vi "Format View Parameter.vi"(9 "Column":T1, 11 "VI Data":T2) -> (2 "View Parameter":string)   [LabVIEW 2020, in "VI Properties Editor.lvlib"]
doc: "Formats the parameter specified by <B>Column</B> into a string value to be used in filter and sort functions."
uses:
  VI Properties Editor.lvlib
  CTLs/VI Data.ctl
  CTLs/VI Properties.ctl
  <vilib>/picture/picture.llb/imagedata.ctl
  CTLs/Control Properties.ctl
  CTLs/Column Name.ctl
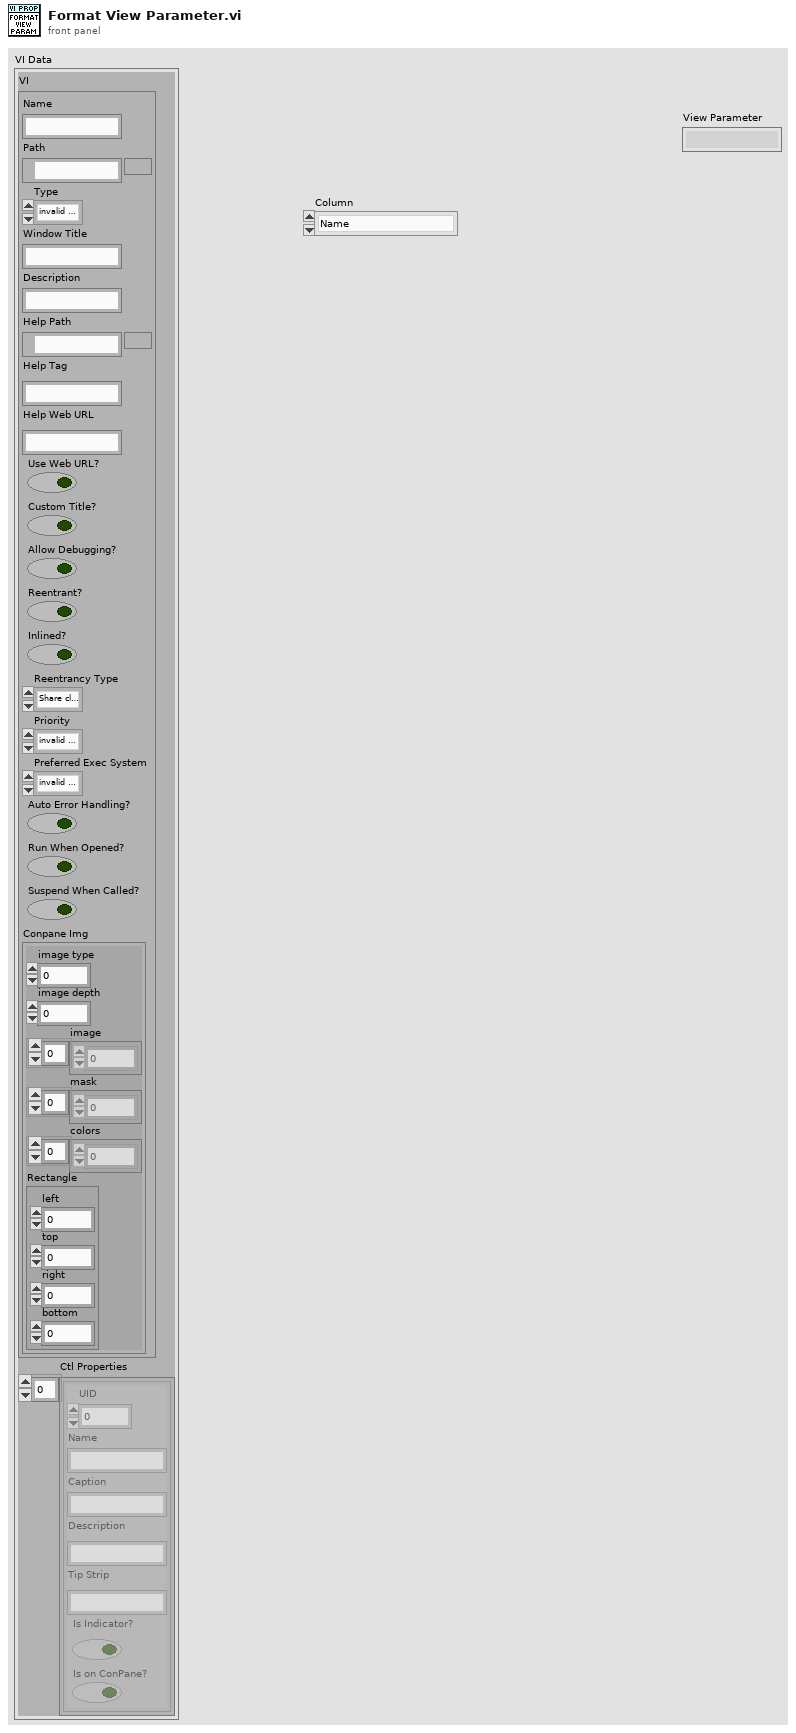
[diagram p1: front panel]
types:
  T1 = typedef "VI Properties Editor.lvlib/Column Name.ctl" = enum16{"Name", "Path", "Type", "Window Title", "Description", "Help Path", "Help Tag", "Custom Title?", "Reentrancy", "Inlined?", "Help URL", "Help Type", "Allow Debugging?", "Auto Error Handling?", "Run When Opened?", "Suspend When Called?", "Priority", "Preferred Exec Sytem"}
  T2 = typedef "VI Properties Editor.lvlib/VI Data.ctl" = cluster{"VI":T3, "Ctl Properties":T5[]}
  T3 = typedef "VI Properties Editor.lvlib/VI Properties.ctl" = cluster{"Name":string, "Path":path, "Type":enum32{"invalid VI type", "Standard VI", "Control VI", "Global VI", "Polymorphic VI", "Configuration VI", "SubSystem", "Facade VI", "Method VI", "Statechart Diagram VI"}, "Window Title":string, "Description":string, "Help Path":path, "Help Tag":string, "Help Web URL":string, "Use Web URL?":bool, "Custom Title?":bool, "Allow Debugging?":bool, "Reentrant?":bool, "Inlined?":bool, "Reentrancy Type":enum16{"Share clones between instances", "Preallocate clone for each instance"}, "Priority":enum32{"invalid priority", "background priority", "normal priority", "above normal priority", "high priority", "time critical priority", "subroutine"}, "Preferred Exec System":enum32{"invalid execution system", "user interface", "standard", "instrument i/o", "data acquisition", "other 1", "other 2", "same as caller"}, "Auto Error Handling?":bool, "Run When Opened?":bool, "Suspend When Called?":bool, "Conpane Img":T4}
  T4 = typedef "imagedata.ctl" = cluster{"image type":i32, "image depth":i32, "image":u8[], "mask":u8[], "colors":u32[], "Rectangle":cluster{"left":i16, "top":i16, "right":i16, "bottom":i16}}
  T5 = typedef "VI Properties Editor.lvlib/Control Properties.ctl" = cluster{"UID":i32, "Name":string, "Caption":string, "Description":string, "Tip Strip":string, "Is Indicator?":bool, "Is on ConPane?":bool}
  T6 = enum32{"invalid VI type", "Standard VI", "Control VI", "Global VI", "Polymorphic VI", "Configuration VI", "SubSystem", "Facade VI", "Method VI", "Statechart Diagram VI"}
  T7 = enum16{"Share clones between instances", "Preallocate clone for each instance"}
  T8 = enum32{"invalid priority", "background priority", "normal priority", "above normal priority", "high priority", "time critical priority", "subroutine"}
  T9 = enum32{"invalid execution system", "user interface", "standard", "instrument i/o", "data acquisition", "other 1", "other 2", "same as caller"}
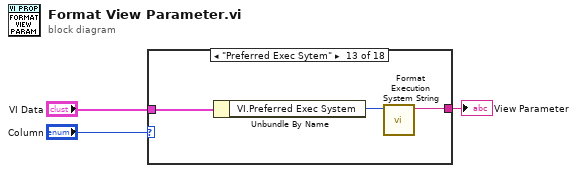
[diagram p0: block diagram]
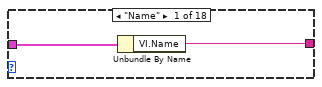
[diagram p2: hidden frame]
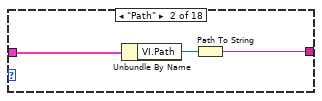
[diagram p3: hidden frame]
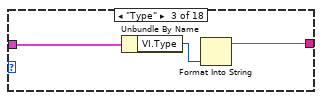
[diagram p4: hidden frame]
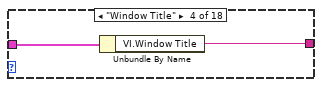
[diagram p5: hidden frame]
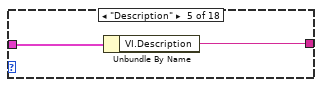
[diagram p6: hidden frame]
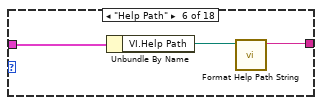
[diagram p7: hidden frame]
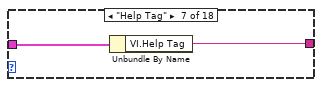
[diagram p8: hidden frame]
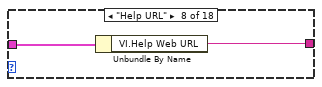
[diagram p9: hidden frame]
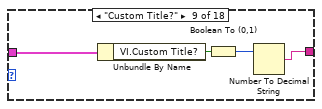
[diagram p10: hidden frame]
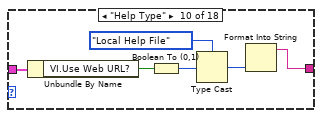
[diagram p11: hidden frame]
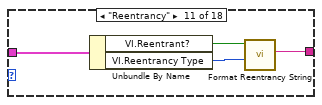
[diagram p12: hidden frame]
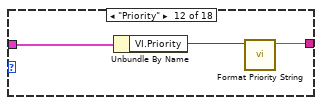
[diagram p13: hidden frame]
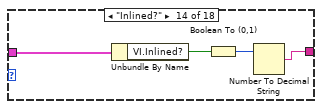
[diagram p14: hidden frame]
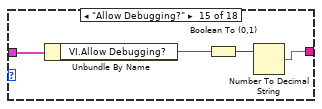
[diagram p15: hidden frame]
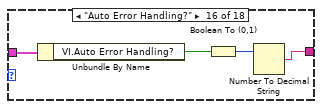
[diagram p16: hidden frame]
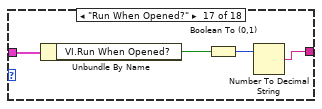
[diagram p17: hidden frame]
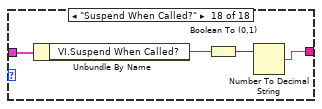
[diagram p18: hidden frame]
diagram:
  n1 = case shown="\"Preferred Exec Sytem\"" "Column" {
    tunnel: "VI Data" -> [w5 w8 w11 w13 w15 w18 w20 w22 w26 w32 w36 w39 w42 w46 w50 w54 w58 w62]
    tunnel: [w4 w6 w10 w12 w14 w17 w19 w21 w23 w27 w34 w38 w40 w43 w47 w51 w55 w59] -> w1
    frame "Name" {
      n2 = Unbundle By Name(w5) -> ("VI.Name"=w4:string)
    }
    frame "Path" {
      n3 = Unbundle By Name(w8) -> ("VI.Path"=w7:path)
      n4 = Path To String(path=w7) -> (string=w6:string)
    }
    frame "Type" {
      n5 = Unbundle By Name(w11) -> ("VI.Type"=w9:T6)
      n6 = Format Into String(w9) -> (resulting string=w10:string)  [unwired: 3 in, 1 out]
    }
    frame "Window Title" {
      n7 = Unbundle By Name(w13) -> ("VI.Window Title"=w12:string)
    }
    frame "Description" {
      n8 = Unbundle By Name(w15) -> ("VI.Description"=w14:string)
    }
    frame "Help Path" {
      n9 = Unbundle By Name(w18) -> ("VI.Help Path"=w16:path)
      n10 = call "Format Help Path String.vi"("Help Path"=w16) -> ("Help Path String"=w17:string)  [unwired: 10 in]
    }
    frame "Help Tag" {
      n11 = Unbundle By Name(w20) -> ("VI.Help Tag"=w19:string)
    }
    frame "Help URL" {
      n12 = Unbundle By Name(w22) -> ("VI.Help Web URL"=w21:string)
    }
    frame "Custom Title?" {
      n13 = Unbundle By Name(w26) -> ("VI.Custom Title?"=w25:bool)
      n14 = Boolean To (0,1)(Boolean=w25) -> (0, 1=w24:i16)
      n15 = Number To Decimal String(number=w24) -> (decimal integer string=w23:string)  [unwired: 1 in]
    }
    frame "Help Type" {
      n16 = Unbundle By Name(w32) -> ("VI.Use Web URL?"=w31:bool)
      n17 = Boolean To (0,1)(Boolean=w31) -> (0, 1=w30:i16)
      n18 = Type Cast(type=enum16{"Local Help File", "Web-based Help"}."Local Help File" ("FP.Help Type"), x=w30) -> (*(type *) &x=w28:enum16{"Local Help File", "Web-based Help"})
      n19 = Format Into String(w28) -> (resulting string=w27:string)  [unwired: 3 in, 1 out]
    }
    frame "Reentrancy" {
      n20 = Unbundle By Name(w36) -> ("VI.Reentrant?"=w33:bool, "VI.Reentrancy Type"=w35:T7)
      n21 = call "Format Reentrancy String.vi"("Reentrancy Type"=w35, "Reentrant?"=w33) -> ("Reentrancy String"=w34:string)  [unwired: 9 in]
    }
    frame "Priority" {
      n22 = Unbundle By Name(w39) -> ("VI.Priority"=w37:T8)
      n23 = call "Format Priority String.vi"("Priority"=w37) -> ("Priority String"=w38:string)  [unwired: 10 in]
    }
    frame "Preferred Exec Sytem" {
      n24 = Unbundle By Name(w42) -> ("VI.Preferred Exec System"=w41:T9)
      n25 = call "Format Execution System String.vi"("Preferred Exec System"=w41) -> ("Preferred Exec System String"=w40:string)  [unwired: 10 in]
    }
    frame "Inlined?" {
      n26 = Unbundle By Name(w46) -> ("VI.Inlined?"=w45:bool)
      n27 = Boolean To (0,1)(Boolean=w45) -> (0, 1=w44:i16)
      n28 = Number To Decimal String(number=w44) -> (decimal integer string=w43:string)  [unwired: 1 in]
    }
    frame "Allow Debugging?" {
      n29 = Unbundle By Name(w50) -> ("VI.Allow Debugging?"=w49:bool)
      n30 = Boolean To (0,1)(Boolean=w49) -> (0, 1=w48:i16)
      n31 = Number To Decimal String(number=w48) -> (decimal integer string=w47:string)  [unwired: 1 in]
    }
    frame "Auto Error Handling?" {
      n32 = Unbundle By Name(w54) -> ("VI.Auto Error Handling?"=w53:bool)
      n33 = Boolean To (0,1)(Boolean=w53) -> (0, 1=w52:i16)
      n34 = Number To Decimal String(number=w52) -> (decimal integer string=w51:string)  [unwired: 1 in]
    }
    frame "Run When Opened?" {
      n35 = Unbundle By Name(w58) -> ("VI.Run When Opened?"=w57:bool)
      n36 = Boolean To (0,1)(Boolean=w57) -> (0, 1=w56:i16)
      n37 = Number To Decimal String(number=w56) -> (decimal integer string=w55:string)  [unwired: 1 in]
    }
    frame "Suspend When Called?" {
      n38 = Unbundle By Name(w62) -> ("VI.Suspend When Called?"=w61:bool)
      n39 = Boolean To (0,1)(Boolean=w61) -> (0, 1=w60:i16)
      n40 = Number To Decimal String(number=w60) -> (decimal integer string=w59:string)  [unwired: 1 in]
    }
  }
  "View Parameter" <- w1
